vi "RunTimeMenu_TCE_RecentInsert.vi"(11 "NewPath":path) -> ()   [LabVIEW 2024]
uses:
  <vilib>/Utility/file.llb/Read Delimited Spreadsheet (string).vi
  <vilib>/Utility/file.llb/Write Delimited Spreadsheet (string).vi
panel:
  out "subarray":string[](array[string])
  out "all rows":string[][](array[string])
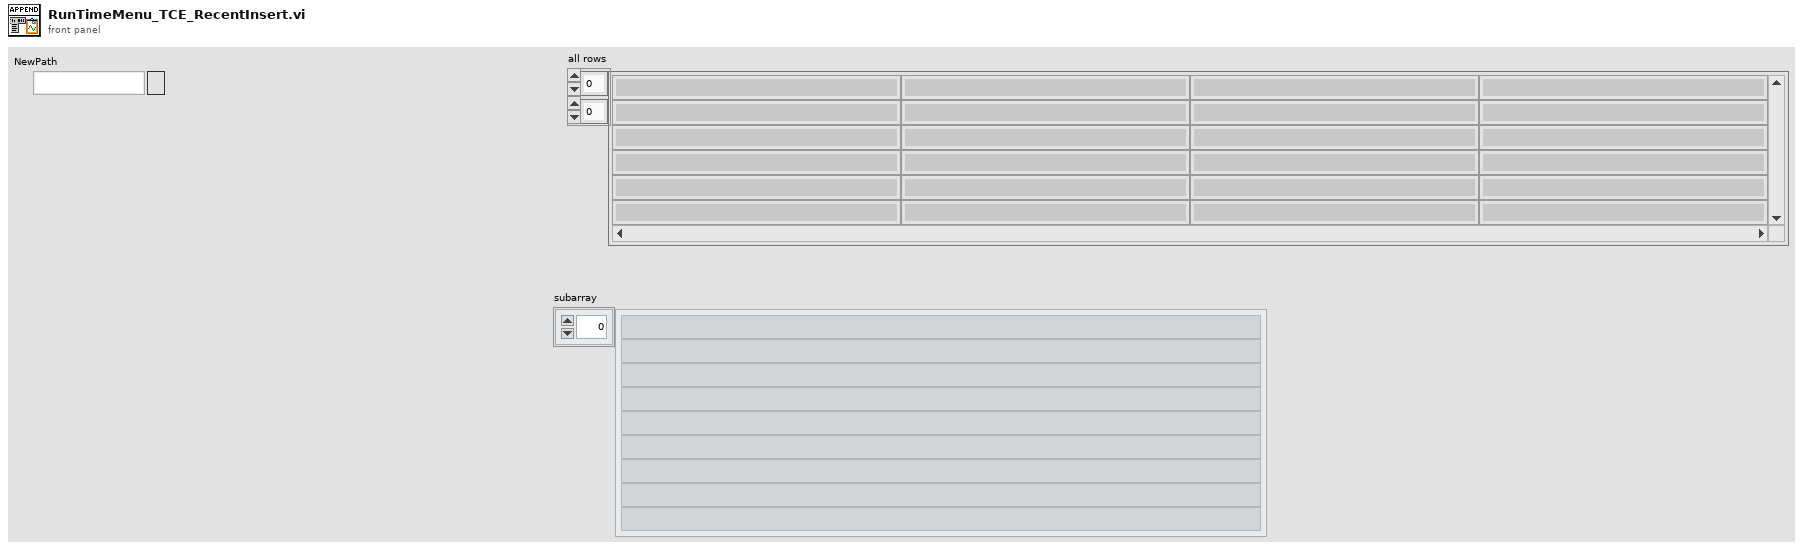
[diagram p1: front panel]
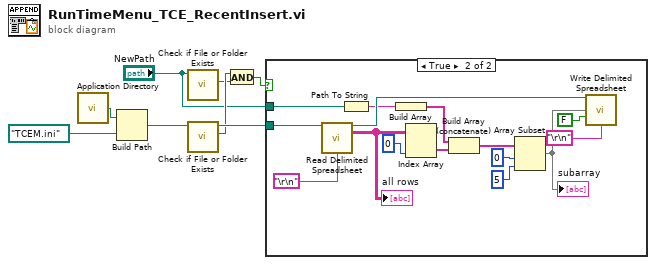
[diagram p0: block diagram]
diagram:
  n1 = call <vilib>:"Application Directory.vi"() -> ("Application Directory"=w8:path)
  n2 = Build Path(base path=w8, name or relative path=path "TCEM.ini") -> (appended path=w6:path)
  n3 = call <vilib>:"Check if File or Folder Exists.vi"("path"="NewPath") -> ("file or folder exists?"=w2:bool)  [unwired: 8 in, 2 out]
  n4 = call <vilib>:"Check if File or Folder Exists.vi"("path"=w6) -> ("file or folder exists?"=w4:bool, "dup path"=w5:path)  [unwired: 8 in, 1 out]
  n5 = And(x=w4, y=w2) -> (x .and. y?=w3:bool)
  n6 = case shown="True" w3 {
    tunnel: w5 -> [_ w20]
    tunnel: "NewPath" -> [_ w10]
    frame False {
    }
    frame True {
      n7 = call-poly <vilib>:"Read Delimited Spreadsheet.vi"("file path (dialog if empty)"=w20, "delimiter (\\t)"="\r\n") -> ("new file path (Not A Path if cancelled)"=w16:path, "all rows"=w23:string[][])  [unwired: 8 in, 4 out]
      "all rows" <- w23
      n8 = Path To String(path=w10) -> (string=w9:string)
      n9 = Build Array(w9) -> (w18:string[])
      n10 = Index Array(array=w23, index (col)=0 ("disabled index (col)")) -> (element=w19:string[])  [unwired: 1 in]
      n11 = Build Array (concatenate)(w18, w19) -> (w17:string[])
      n12 = Array Subset(array=w17, index=0, length=5) -> (w14:string[])
      "subarray" <- w14
      n13 = call-poly <vilib>:"Write Delimited Spreadsheet.vi"("file path (dialog if empty)"=w16, "1D data"=w14, "append to file? (new file:F)"=FALSE, "delimiter (\\t)"="\r\n") -> ()  [unwired: 10 in, 2 out]
    }
  }
